vi "回原点运动.vi"() -> ()   [LabVIEW 2011]
uses:
  <userlib>/LTDMC/LTDMC.lvlib
panel:
  in  "停止速度":dbl=100.0
  in  "org_logic":u16(ring) items=["低电平有效", "高电平有效"]
  in  "vel_mode":u16(ring) items=["低速回原点", "高速回原点"]
  in  "home_dir":u16(ring) items=["负方向回原点", "正方向回原点"]
  in  "home_mode":u16(ring) items=["一次回零", "一次回零加反找", "二次回零", "一次回零加EZ一次回零"]
  out "运行时间":dbl
  out "当前状态":string
  out "当前速度":dbl
  out "当前位置":i32
  out "运行曲线图":cluster{dbl[], dbl[]}[](graph)
  in  "减速时间":dbl=0.5
  in  "加速时间":dbl=0.5
  in  "运行速度":dbl=1000.0
  in  "起始速度":dbl=200.0
  in  "退出":bool
  in  "紧急停止":bool
  in  "减速停止":bool
  in  "运行":bool
  in  "轴号选择":enum32{"X轴", "Y轴", "Z轴", "C轴"}(radio)
  in  "脉冲清零":bool
  in  "卡号选择":u16(ring) items=["0"]
  out "init":bool
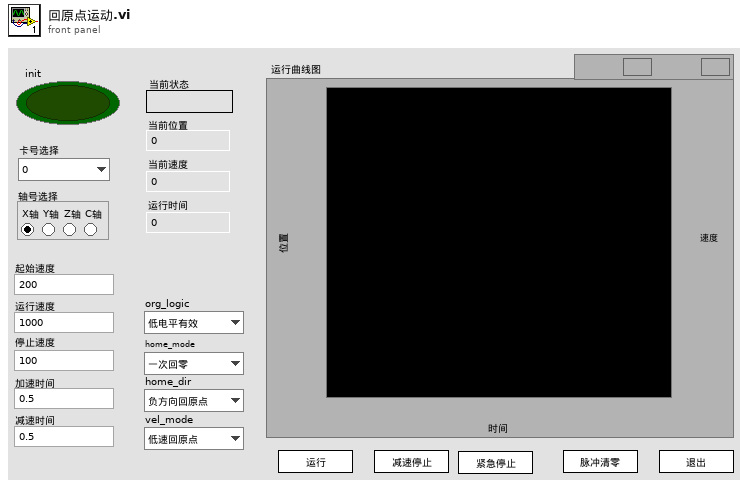
[diagram p1: front panel]
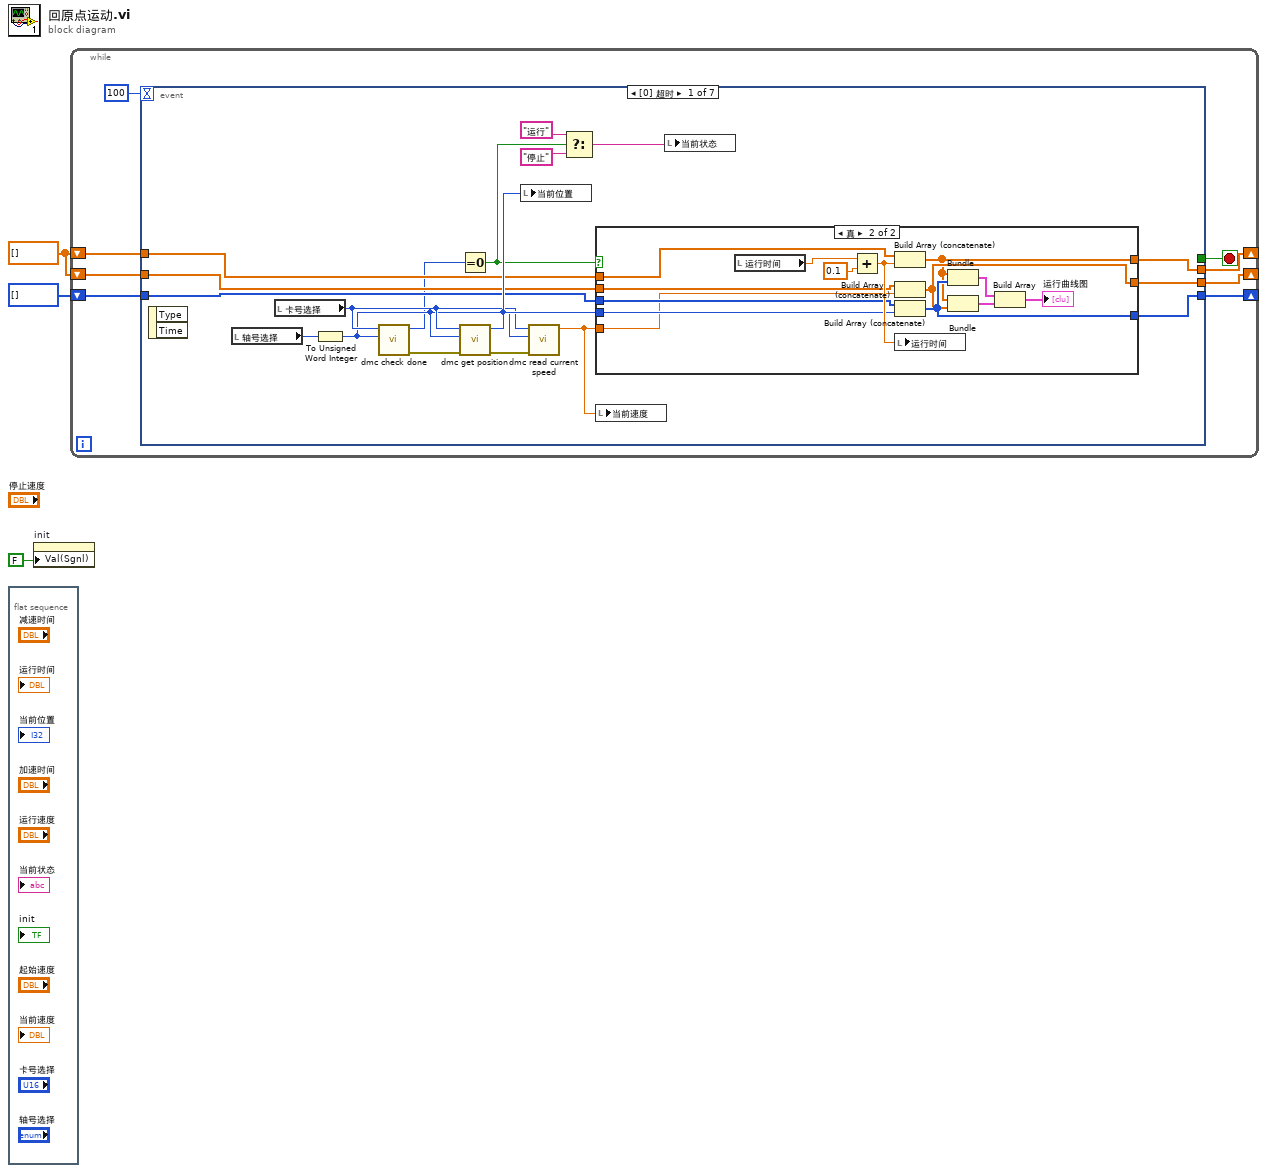
[diagram p0: block diagram]
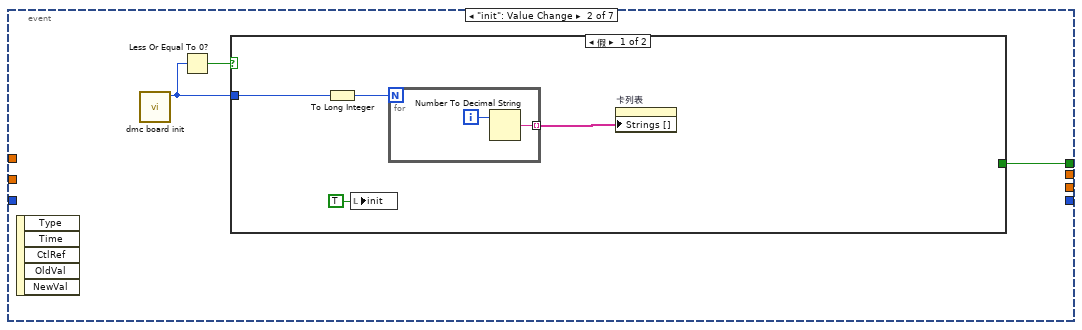
[diagram p3: hidden frame]
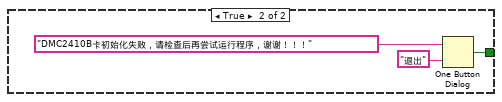
[diagram p4: hidden frame]
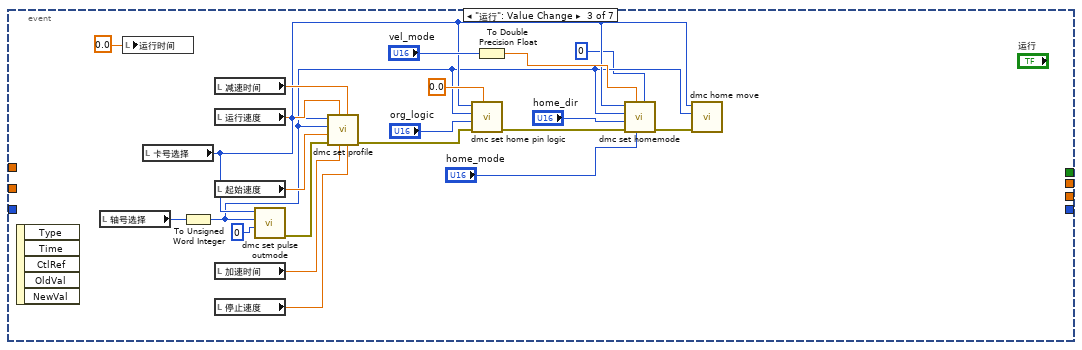
[diagram p5: hidden frame]
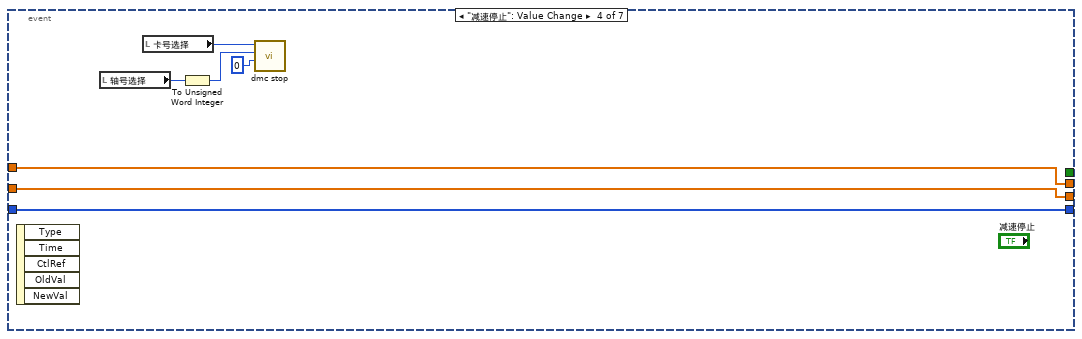
[diagram p6: hidden frame]
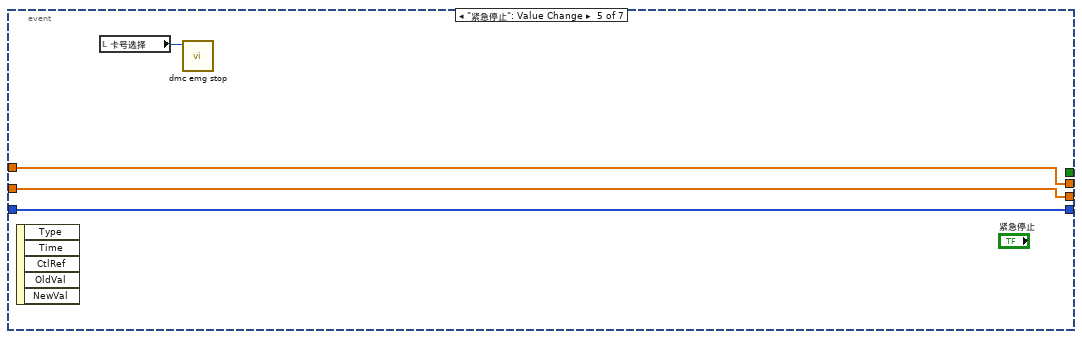
[diagram p7: hidden frame]
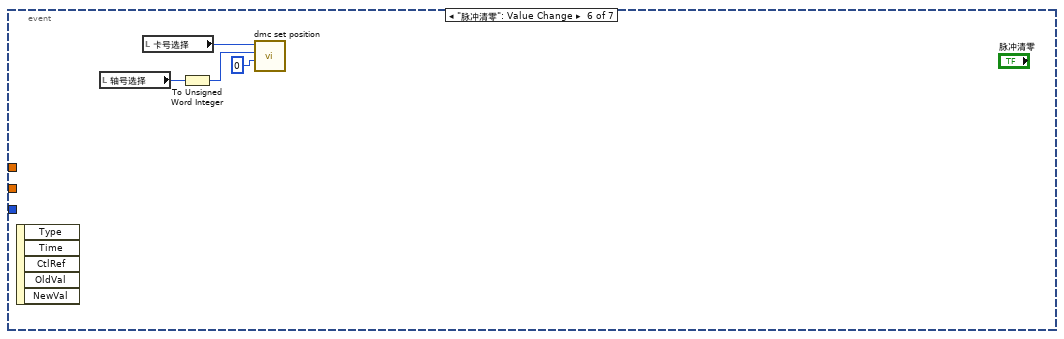
[diagram p8: hidden frame]
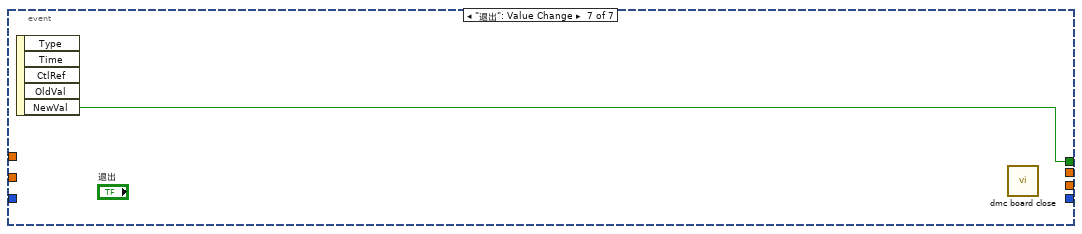
[diagram p9: hidden frame]
diagram:
  w1 = dbl[] []
  n1 = flat-sequence {
    frame #0 {
    }
  }
  n2 = property on="init" class="Bool (严格)"("Val(Sgnl)"=FALSE ("值(信号)")) -> ()  [unwired: 2 in, 2 out]
  n3 = while {
    shift-right: [w9] -> _
    shift-left: w1 -> [w8]
    shift-right: [w7] -> _
    shift-left: i32[] [] -> [w6]
    shift-right: [w4] -> _
    shift-left: w1 -> [w5]
    stop <- w11 stop-if-true
    n4 = event shown="[0] 超时" {
      selector: _ -> [_ _ _ _ _ _ _]
      dyn-events: _ -> [_ _ _ _ _ _ _]
      timeout: 100 -> [_ _ _ _ _ _ _]
      tunnel: [_ w45 _ _ _ _ w92] -> w11
      tunnel: [w24 _ _ w82 w87 _ _] -> w9
      tunnel: w8 -> [w23 _ _ w82 w87 _ _]
      tunnel: [w22 _ _ w81 w86 _ _] -> w7
      tunnel: w6 -> [w21 _ _ w81 w86 _ _]
      tunnel: w5 -> [w20 _ _ w80 w85 _ _]
      tunnel: [w19 _ _ w80 w85 _ _] -> w4
      event Timeout {
        n5 = event-data() -> ()  [unwired: 1 in, 2 out]
        n6 = local read "轴号选择"() -> (w29:enum32{"X轴", "Y轴", "Z轴", "C轴"})
        n7 = local read "卡号选择"() -> (w15:u16)
        n8 = To Unsigned Word Integer(number=w29) -> (unsigned 16bit integer=w14:u16)
        n9 = call "dmc check done.vi"("axis"=w14, "CardNo"=w15) -> ("error out"=w16:errorcluster, "function return"=w12:i16)  [unwired: 8 in]
        n10 = Equal To 0?(x=w12) -> (x = 0?=w17:bool)
        n11 = call "dmc get position.vi"("error in (no error)"=w16, "axis"=w14, "CardNo"=w15) -> ("error out"=w13:errorcluster, "function return"=w25:i32)  [unwired: 7 in]
        n12 = local write "当前位置"(w25) -> ()
        n13 = call "dmc read current speed.vi"("error in (no error)"=w13, "axis"=w14, "CardNo"=w15) -> ("function return"=w18:dbl)  [unwired: 7 in, 1 out]
        n14 = Select(t="运行" ("当前状态"), s=w17, f="停止" ("当前状态")) -> (s? t:f=w28:string)
        n15 = case shown="真" w17 {
          tunnel: w25 -> [_ w39]
          tunnel: [_ w33] -> w24
          tunnel: w23 -> [_ w40]
          tunnel: [_ w37] -> w22
          tunnel: w21 -> [_ w38]
          tunnel: w20 -> [_ w36]
          tunnel: [_ w34] -> w19
          tunnel: w18 -> [_ w35]
          frame False {
          }
          frame True {
            n16 = local read "运行时间"() -> (w43:dbl)
            n17 = Add(x=w43, y=0.1) -> (x+y=w41:dbl)
            n18 = Build Array (concatenate)(w40, w41) -> (w33:dbl[])
            n19 = Build Array (concatenate)(w36, w35) -> (w34:dbl[])
            n20 = Build Array (concatenate)(w38, w39) -> (w37:i32[])
            n21 = local write "运行时间"(w41) -> ()
            n22 = Bundle(w33, w37) -> (w31:cluster{dbl[], i32[]})  [unwired: 1 in]
            n23 = Bundle(w33, w34) -> (w32:cluster{dbl[], dbl[]})  [unwired: 1 in]
            n24 = Build Array(w31, w32) -> (→"运行曲线图":cluster{dbl[], dbl[]}[])
          }
        }
        n25 = local write "当前速度"(w18) -> ()
        n26 = local write "当前状态"(w28) -> ()
      }
      event "init": Value Change {
        n27 = event-data() -> ()  [unwired: 1 in, 5 out]
        n28 = call "dmc board init.vi"() -> ("function return"=w44:i16)  [unwired: 10 in, 1 out]
        n29 = Less Or Equal To 0?(x=w44) -> (x <= 0?=w46:bool)
        n30 = case shown="假" w46 {
          tunnel: [_ w53] -> w45
          tunnel: w44 -> [w50 _]
          frame False {
            n31 = To Long Integer(number=w50) -> (32bit integer=w49:i32)
            n32 = local write "init"(TRUE ("init")) -> ()
            n33 = for {
              N: w49 -> [_]
              tunnel: [w51] -> w48 mode=indexing
              i -> [w52]
              n34 = Number To Decimal String(number=w52) -> (decimal integer string=w51:string)  [unwired: 1 in]
            }
            n35 = property on="卡列表" class="Ring (严格)"("Strings []"=w48) -> ()  [unwired: 2 in, 2 out]
          }
          frame True {
            n36 = One Button Dialog(message="DMC2410B卡初始化失败，请检查后再尝试运行程序，谢谢！！！" ("消息"), button name ("OK")="退出" ("按钮名称（“确定”）")) -> (true=w53:bool)
          }
        }
      }
      event "运行": Value Change {
        n37 = event-data() -> ()  [unwired: 1 in, 5 out]
        n38 = local read "轴号选择"() -> (w76:enum32{"X轴", "Y轴", "Z轴", "C轴"})
        n39 = local write "运行时间"(0.0 ("运行时间")) -> ()
        n40 = local read "卡号选择"() -> (w62:u16)
        n41 = To Unsigned Word Integer(number=w76) -> (unsigned 16bit integer=w61:u16)
        n42 = local read "减速时间"() -> (w64:dbl)
        n43 = local read "运行速度"() -> (w72:dbl)
        n44 = local read "起始速度"() -> (w73:dbl)
        n45 = local read "加速时间"() -> (w71:dbl)
        n46 = local read "停止速度"() -> (w66:dbl)
        n47 = call "dmc set pulse outmode.vi"("outmode"=u16 0, "axis"=w61, "CardNo"=w62) -> ("error out"=w59:errorcluster)  [unwired: 7 in, 1 out]
        n48 = call "dmc set profile.vi"("stop_vel"=w66, "Tdec"=w64, "Tacc"=w71, "Max_Vel"=w72, "error in (no error)"=w59, "Min_Vel"=w73, "axis"=w61, "CardNo"=w62) -> ("error out"=w56:errorcluster)  [unwired: 2 in, 1 out]
        n49 = call "dmc set home pin logic.vi"("filter"=0.0, "error in (no error)"=w56, "org_logic"="org_logic", "axis"=w61, "CardNo"=w62) -> ("error out"=w58:errorcluster)  [unwired: 5 in, 1 out]
        n50 = To Double Precision Float(number="vel_mode") -> (double precision float=w63:dbl)
        n51 = call "dmc set homemode.vi"("EZ_count"=u16 0, "mode"="home_mode", "vel_mode"=w63, "error in (no error)"=w58, "home_dir"="home_dir", "axis"=w61, "CardNo"=w62) -> ("error out"=w57:errorcluster)  [unwired: 3 in, 1 out]
        n52 = call "dmc home move.vi"("error in (no error)"=w57, "axis"=w61, "CardNo"=w62) -> ()  [unwired: 7 in, 2 out]
      }
      event "减速停止": Value Change {
        n53 = event-data() -> ()  [unwired: 1 in, 5 out]
        n54 = local read "轴号选择"() -> (w83:enum32{"X轴", "Y轴", "Z轴", "C轴"})
        n55 = local read "卡号选择"() -> (w78:u16)
        n56 = To Unsigned Word Integer(number=w83) -> (unsigned 16bit integer=w77:u16)
        n57 = call "dmc stop.vi"("stop_mode"=u16 0, "axis"=w77, "CardNo"=w78) -> ()  [unwired: 7 in, 2 out]
      }
      event "紧急停止": Value Change {
        n58 = event-data() -> ()  [unwired: 1 in, 5 out]
        n59 = local read "卡号选择"() -> (w84:u16)
        n60 = call "dmc emg stop.vi"("CardNo"=w84) -> ()  [unwired: 9 in, 2 out]
      }
      event "脉冲清零": Value Change {
        n61 = event-data() -> ()  [unwired: 1 in, 5 out]
        n62 = local read "轴号选择"() -> (w91:enum32{"X轴", "Y轴", "Z轴", "C轴"})
        n63 = local read "卡号选择"() -> (w88:u16)
        n64 = To Unsigned Word Integer(number=w91) -> (unsigned 16bit integer=w89:u16)
        n65 = call "dmc set position.vi"("current_position"=0, "axis"=w89, "CardNo"=w88) -> ()  [unwired: 7 in, 2 out]
      }
      event "退出": Value Change {
        n66 = event-data() -> ("NewVal"=w92:bool)  [unwired: 1 in, 4 out]
        n67 = call "dmc board close.vi"() -> ()  [unwired: 10 in, 2 out]
      }
    }
  }
